vi "Update Template for Spartan 5.0.vi"(7 "Connection Refnum":T1, 8 "error in (no error)":errorcluster, 9 "EncodedParameters":string, 10 "Old Template Record":T6, 11 "All Fields":T3[](array[typedef])) -> (0 "error out":errorcluster, 1 "(key,values)":T2, 2 "New Template Record":T6, 5 "Connection Refnum 2":T1)   [LabVIEW 2011]
uses:
  Template Record.ctl
  Fields/Field Record.ctl
  Fields/Field DataTypes.ctl
  Fields/Field NextItem.ctl
  ITK EXT/utils/keyedarr.llb/Keyed Array.ctl
  Summitek EXT/ODBC/SQL Controls/Connection Refnum.ctl
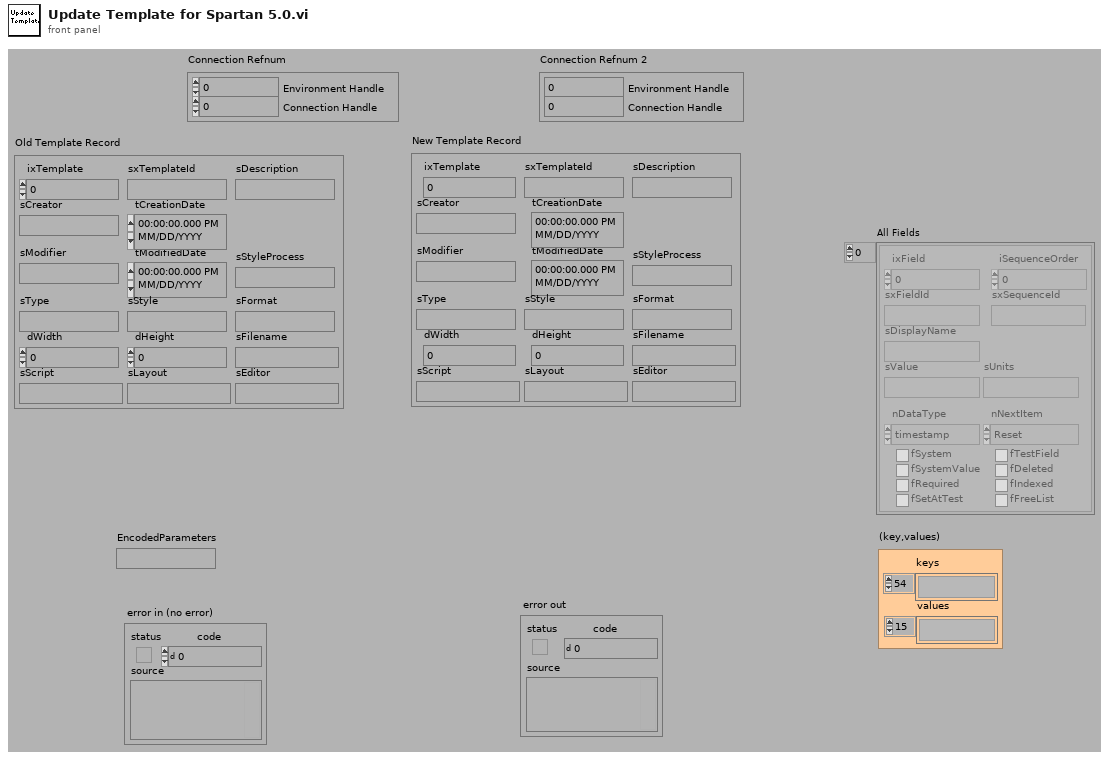
[diagram p1: front panel]
types:
  T1 = typedef "Connection Refnum.ctl" = cluster{"Environment Handle":i32, "Connection Handle":i32}
  T2 = typedef "Keyed Array.ctl" = cluster{"keys":string[], "values":string[]}
  T3 = typedef "Field Record.ctl" = cluster{"ixField":i32, "iSequenceOrder":i32, "sxFieldId":string, "sxSequenceId":string, "sDisplayName":string, "sValue":string, "sUnits":string, "nDataType":T4, "nNextItem":T5, "fSystem":bool, "fSystemValue":bool, "fRequired":bool, "fSetAtTest":bool, "fTestField":bool, "fDeleted":bool, "fIndexed":bool, "fFreeList":bool}
  T4 = typedef "Field DataTypes.ctl" = enum32{"text", "numeric", "list", "timestamp", "boolean"}
  T5 = typedef "Field NextItem.ctl" = enum32{"Reset", "Retain", "Auto-Increment"}
  T6 = typedef "Template Record.ctl" = cluster{"ixTemplate":i32, "sxTemplateId":string, "sDescription":string, "sCreator":string, "tCreationDate":timestamp, "sModifier":string, "tModifiedDate":timestamp, "sType":string, "sStyle":string, "sFormat":string, "dWidth":dbl, "dHeight":dbl, "sFilename":string, "sScript":string, "sLayout":string, "sEditor":string, "sStyleProcess":string}
  T7 = cluster{"sFilename":string, "sScript":string, "sLayout":string, "sEditor":string}
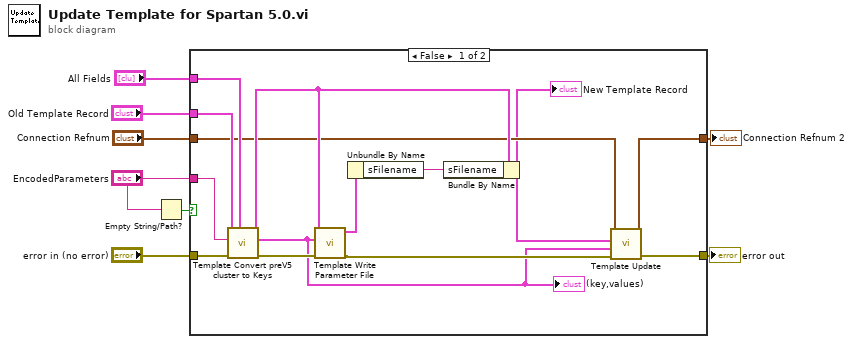
[diagram p0: block diagram]
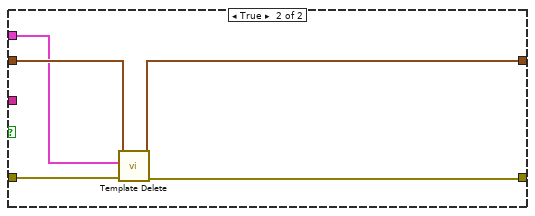
[diagram p2: hidden frame]
diagram:
  n1 = Empty String/Path?(string/path="EncodedParameters") -> (empty?=w3:bool)
  n2 = case shown="False" w3 {
    tunnel: [w11 w26] -> w8
    tunnel: "error in (no error)" -> [w22 w27]
    tunnel: "EncodedParameters" -> [w18 _]
    tunnel: "Old Template Record" -> [w17 w24]
    tunnel: "All Fields" -> [w15 _]
    tunnel: "Connection Refnum" -> [w13 w25]
    tunnel: [w12 w23] -> w1
    frame False {
      n3 = call "Template Convert preV5 cluster to Keys.vi"("ALL Fields"=w15, "error in (no error)"=w22, "EncodedParameters"=w18, "Old Template Record"=w17) -> ("error out"=w21:errorcluster, "(key,values)"=w9:T2, "New Template Record"=w16:T6)  [unwired: 5 out]
      "(key,values)" <- w9
      n4 = call "Template Write Parameter File.vi"("error in (no error)"=w21, "Parameters (empty)"=w9, "Template Record"=w16) -> ("error out"=w14:errorcluster, "Files"=w20:T7)  [unwired: 2 in, 5 out]
      n5 = Unbundle By Name(w20) -> ("sFilename"=w19:string)
      n6 = Bundle By Name(cluster=w16, "sFilename"=w19) -> (w10:T6)
      "New Template Record" <- w10
      n7 = call "Template Update.vi"("error in (no error)"=w14, "Parameters (empty)"=w9, "Template Record"=w10, "Connection Refnum"=w13) -> ("error out"=w11:errorcluster, "Connection Refnum"=w12:T1)  [unwired: 6 out]
    }
    frame True {
      n8 = call "Template Delete.vi"("error in (no error)"=w27, "Template Record"=w24, "Connection Refnum"=w25) -> ("error out"=w26:errorcluster, "Connection Refnum"=w23:T1)  [unwired: 7 out]
    }
  }
  "error out" <- w8
  "Connection Refnum 2" <- w1
